vi "table to spreadsheet with labels.vi"(10 "format string":string="%g", 11 "lookup table":T1(array[cluster])) -> (3 "spreadsheet table":string)   [LabVIEW 2013]
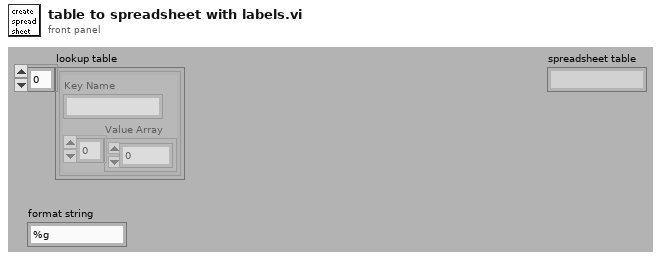
[diagram p1: front panel]
types:
  T1 = cluster{"Key Name":string, "Value Array":dbl[]}[]
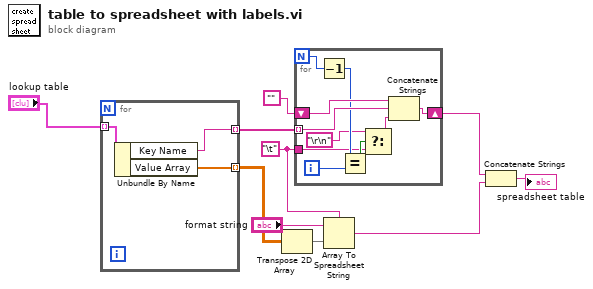
[diagram p0: block diagram]
diagram:
  w7 = "\t"
  n1 = for {
    tunnel: "lookup table" -> [w13] mode=indexing
    tunnel: [w12] -> w9 mode=indexing
    tunnel: [w11] -> w6 mode=indexing
    n2 = Unbundle By Name(w13) -> ("Key Name"=w12:string, "Value Array"=w11:dbl[])
  }
  n3 = Transpose 2D Array(2D array=w6) -> (transposed array=w2:dbl[][])
  n4 = for {
    N -> [w19]
    tunnel: w9 -> [w23] mode=indexing
    shift-right: [w22] -> w4
    shift-left: "" -> [w21]
    tunnel: w7 -> [w16]
    i -> [w20]
    n5 = Decrement(x=w19) -> (x-1=w18:i32)
    n6 = Equal?(x=w18, y=w20) -> (x = y?=w17:bool)
    n7 = Select(t="\r\n", s=w17, f=w16) -> (s? t:f=w15:string)
    n8 = Concatenate Strings(w21, w23, w15) -> (w22:string)
  }
  n9 = Array To Spreadsheet String(delimiter (Tab)=w7, array=w2, 3:"format string") -> (spreadsheet string=w1:string)
  n10 = Concatenate Strings(w4, w1) -> (→"spreadsheet table":string)
